vi "RTM - Add Unbound Channels.vi"(8 "error in (no error)":errorcluster, 11 "Node Ptr":T1 format="%.0x") -> (0 "error out":errorcluster)   [LabVIEW 2016, in "UDP-Custom-Device System Explorer.lvlib"]
uses:
  UDP-Custom-Device System Explorer.lvlib
  <vilib>/NI Veristand/Custom Device API/Custom Device Item Ref.ctl
  Types/Channel Data Type.ctl
  <vilib>/NI Veristand/Custom Device API/Custom Device Channel.ctl
  <vilib>/NI Veristand/Custom Device API/Custom Device Channel Type.ctl
  Shared/Constants.vi
  <vilib>/NI VeriStand/Custom Device API/Custom Device API.lvlib
  Shared/UDP-Custom-Device Shared.lvlib
  <vilib>/NI VeriStand/Custom Device Tools/Custom Device Utility Library/Custom Device Utility Library.lvlib
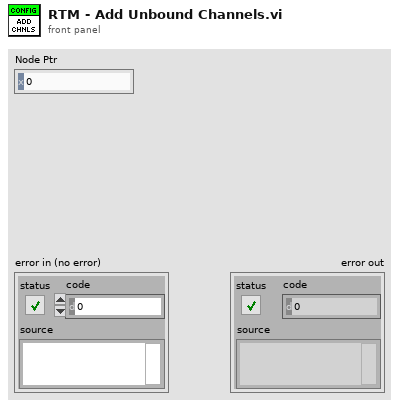
[diagram p1: front panel]
types:
  T1 = typedef "Custom Device API.lvlib/Custom Device Item Ref.ctl" = u64
  T2 = typedef "Custom Device API.lvlib/Custom Device Channel.ctl" = cluster{"Type":T3, "Units":string, "Default Value":dbl, "Faultable":bool, "Scalable":bool}
  T3 = typedef "Custom Device API.lvlib/Custom Device Channel Type.ctl" = enum16{"Input", "Output"}
  T4 = typedef "UDP-Custom-Device Shared.lvlib/Channel Data Type.ctl" = enum16{"Boolean", "Single"}
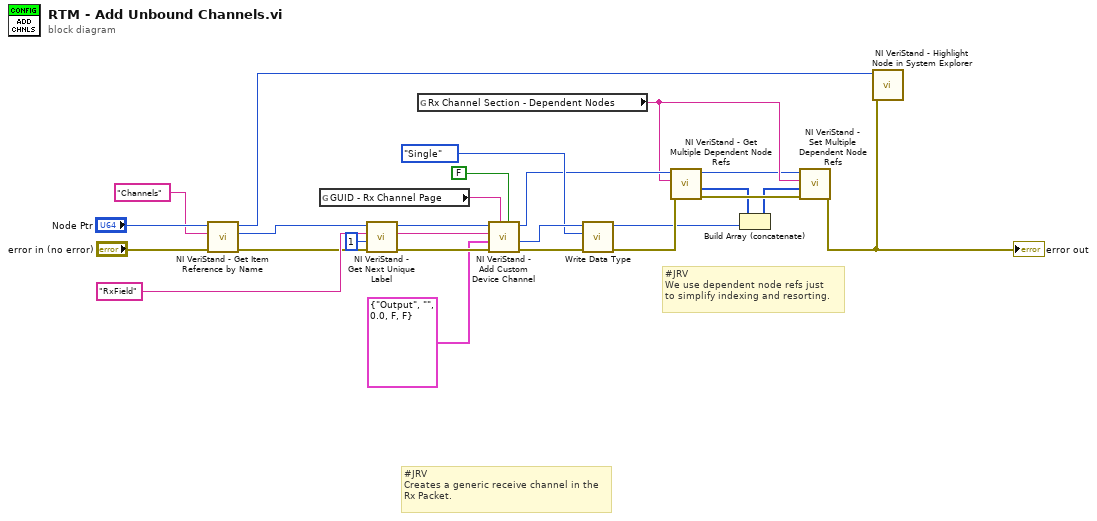
[diagram p0: block diagram]
diagram:
  # "#JRV\nWe use dependent node refs just\nto simplify indexing and resorting."
  # "#JRV\nCreates a generic receive channel in the \nRx Packet."
  n1 = call <vilib>:"NI VeriStand - Get Item Reference by Name.vi"("error in (no error)"="error in (no error)", "Item Name"="Channels" ("Section Name"), "Parent Ref in"="Node Ptr") -> ("error out"=w12:errorcluster, "Item Ref"=w11:T1, "Parent Ref out"=w10:T1)  [unwired: 5 in, 1 out]
  n2 = global read "Constants.vi" "GUID - Rx Channel Page"() -> (w26:string)
  n3 = call <vilib>:"NI VeriStand - Get Next Unique Label.vi"("error in (no error)"=w12, "Start Value (1)"=1, "Label"="RxField", "Parent Ref in"=w11) -> ("error out"=w23:errorcluster, "Label out"=w22:string, "Parent Ref dup"=w21:T1)  [unwired: 4 in, 1 out]
  n4 = global read "Constants.vi" "Rx Channel Section - Dependent Nodes"() -> (w8:string)
  n5 = call <vilib>:"NI VeriStand - Add Custom Device Channel.vi"("Highlight? (F)"=FALSE, "GUID (Default Channel)"=w26, "error in (no error)"=w23, "Channel"=T2 {"Type"=enum."Output", "Units"="", "Default Value"=0.0, "Faultable"=FALSE, "Scalable"=FALSE}, "Channel Name"=w22, "Parent Ref in"=w21) -> ("error out"=w18:errorcluster, "Channel Ref"=w19:T1, "Parent Ref out"=w9:T1)  [unwired: 2 in, 1 out]
  n6 = call "Write Data Type.vi"("error in (no error)"=w18, "Data Type"=Channel_Data_Type."Single", "Node Ptr"=w19) -> ("error out"=w5:errorcluster, "Node Ptr out"=w3:T1)  [unwired: 7 in]
  n7 = call <vilib>:"NI VeriStand - Get Multiple Dependent Node Refs.vi"("error in (no error)"=w5, "Base Property Name"=w8, "Item Ref in"=w9) -> ("error out"=w6:errorcluster, "Dependent Node Refs"=w2:T1[], "Item Ref out"=w7:T1)  [unwired: 6 in]
  n8 = Build Array (concatenate)(w2, w3) -> (w1:T1[])
  n9 = call <vilib>:"NI VeriStand - Set Multiple Dependent Node Refs.vi"("error in (no error)"=w6, "Dependent Node Refs"=w1, "Base Property Name"=w8, "Item Ref in"=w7) -> ("error out"=w4:errorcluster)  [unwired: 6 in, 1 out]
  "error out" <- w4
  n10 = call <vilib>:"NI VeriStand - Highlight Node in System Explorer.vi"("error in (no error)"=w4, "Item Ref in"=w10) -> ()  [unwired: 8 in, 2 out]
